vi "Enumerate Hardware.vi"(8 "error in (no error)":errorcluster, 11 "Hardware Info Module in":refnum<class "Hardware Info Module.lvclass">) -> (0 "error out":errorcluster, 3 "Hardware Info Module out":refnum<class "Hardware Info Module.lvclass">)   [LabVIEW 2023, in "Volatus.lvlib" / "Hardware Info Module.lvclass"]
uses:
  Hardware Info Module.lvclass
  HW Info.ctl
  <vilib>/nisyscfg/Close (Hardware).vi
  <vilib>/nisyscfg/Close (System).vi
  <vilib>/nisyscfg/nisyscfg.lvlib
  <resource>/objmgr/pxisysapi.rc
  <resource>/objmgr/nicriosae.rc
panel:
  out "Array":T1[](array[typedef])
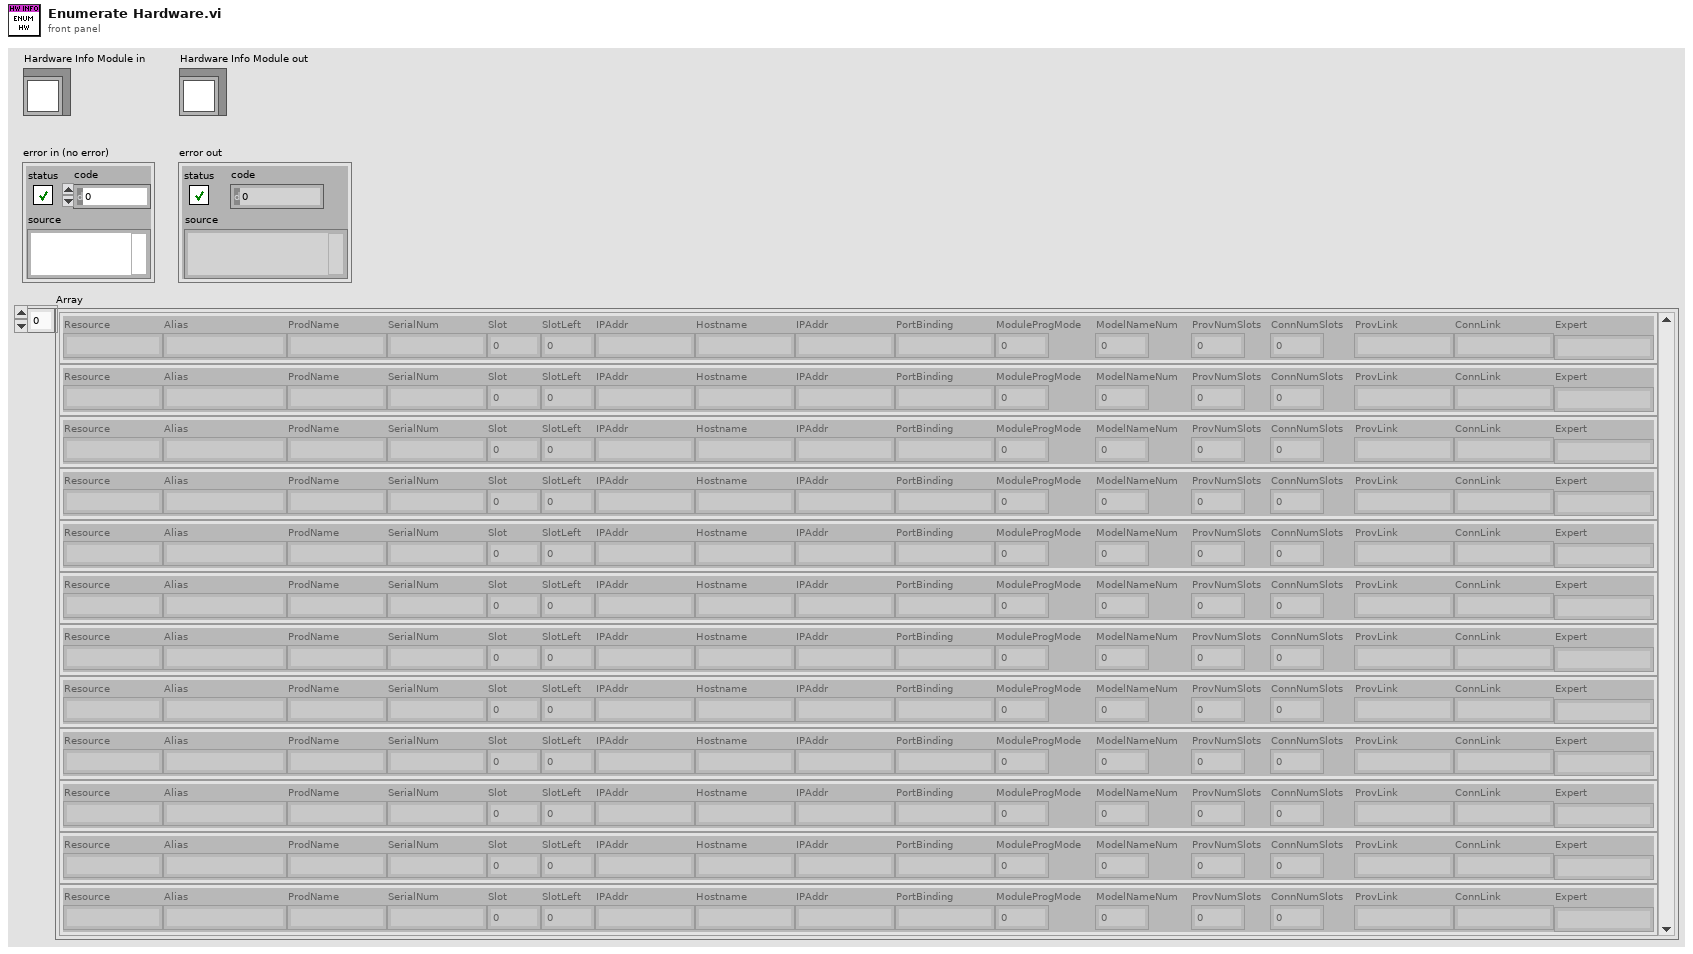
[diagram p1: front panel]
types:
  T1 = typedef "Volatus.lvlib/Hardware Info Module.lvclass/HW Info.ctl" = cluster{"Resource":string, "Alias":string, "ProdName":string, "SerialNum":string, "Slot":i32, "SlotLeft":u32, "IPAddr":string, "Hostname":string, "IPAddr":string, "PortBinding":string, "ModuleProgMode":u32, "ModelNameNum":u32, "ProvNumSlots":i32, "ConnNumSlots":i32, "ProvLink":string, "ConnLink":string, "Expert":string}
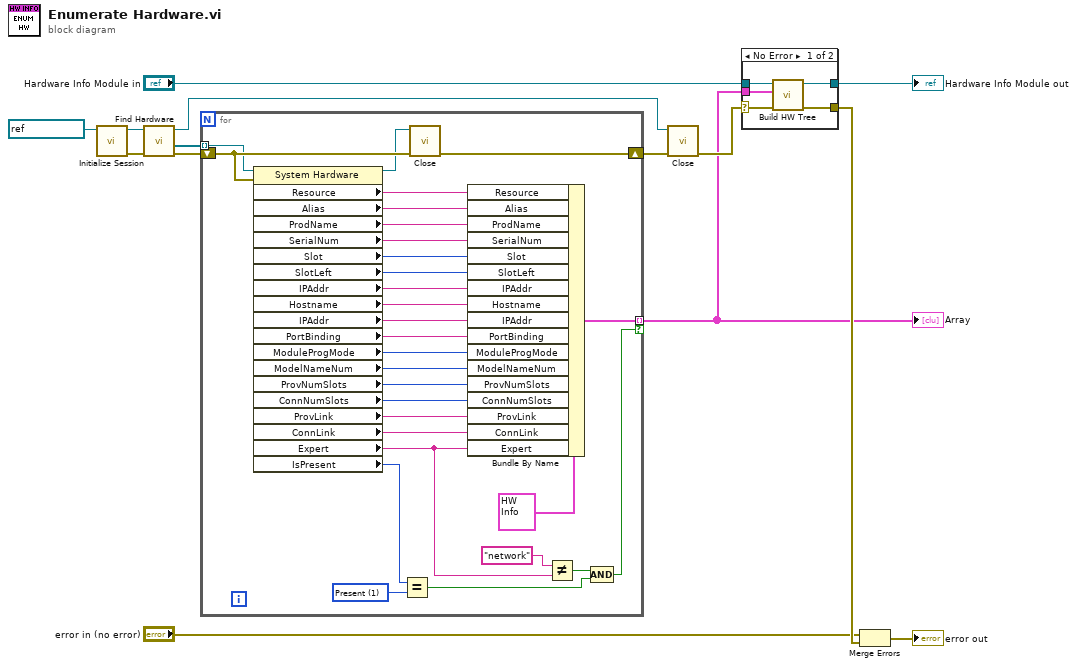
[diagram p0: block diagram]
diagram:
  n1 = call <vilib>:"Initialize Session.vi"("Target (localhost)"=refnum<k21> "localhost") -> ("error out"=w2:errorcluster, "Session out"=w3:refnum<k21>)  [unwired: 9 in]
  n2 = call <vilib>:"Find Hardware.vi"("error in (no error)"=w2, "Session in"=w3) -> ("error out"=w10:errorcluster, "Resources out"=w9:refnum<k20>[], "Session out"=w7:refnum<k21>)  [unwired: 6 in, 1 out]
  n3 = for {
    tunnel: w9 -> [w42] mode=indexing
    tunnel: [w17] -> w5 mode=indexing if=w36
    shift-right: [w34] -> w8
    shift-left: w10 -> [w43]
    w40 = 1 items=["Initializing"=-2, "Unknown"=-1, "Not Present"=0, "Present"=1] ("Devices & Chassis:Is Present")
    n4 = property class="System Hardware"(reference=w42, error in=w43) -> (reference out=w35:refnum<k20>, "Resource"=w16:string, "Alias"=w32:string, "ProdName"=w31:string, "SerialNum"=w30:string, "Slot"=w29:i32, "SlotLeft"=w28:u32, "IPAddr"=w27:string, "Hostname"=w26:string, "IPAddr"=w25:string, "PortBinding"=w24:string, "ModuleProgMode"=w23:u32, "ModelNameNum"=w22:u32, "ProvNumSlots"=w21:i32, "ConnNumSlots"=w20:i32, "ProvLink"=w19:string, "ConnLink"=w18:string, "Expert"=w15:string, "IsPresent"=w41:i32)  [unwired: 1 out]
    n5 = Equal?(x=w41, y=w40) -> (x = y?=w37:bool)
    n6 = call-poly <vilib>:"Close.vi"("error in (no error)"=w43, "Resource in"=w35) -> ("error out"=w34:errorcluster)  [unwired: 9 in]
    n7 = Bundle By Name(cluster=T1 {"Resource"="", "Alias"="", "ProdName"="", "SerialNum"="", "Slot"=0, "SlotLeft"=0, "IPAddr"="", "Hostname"="", "IPAddr"="", "PortBinding"="", "ModuleProgMode"=0, "ModelNameNum"=0, "ProvNumSlots"=0, "ConnNumSlots"=0, "ProvLink"="", "ConnLink"="", "Expert"=""} ("HW Info"), "Resource"=w16, "Alias"=w32, "ProdName"=w31, "SerialNum"=w30, "Slot"=w29, "SlotLeft"=w28, "IPAddr"=w27, "Hostname"=w26, "IPAddr"=w25, "PortBinding"=w24, "ModuleProgMode"=w23, "ModelNameNum"=w22, "ProvNumSlots"=w21, "ConnNumSlots"=w20, "ProvLink"=w19, "ConnLink"=w18, "Expert"=w15) -> (w17:T1)
    n8 = Not Equal?(x="network" ("y"), y=w15) -> (x != y?=w38:bool)
    n9 = Compound Arithmetic op=AND(w38, w37) -> (w36:bool)
  }
  "Array" <- w5
  n10 = call-poly <vilib>:"Close.vi"("error in (no error)"=w8, "Session in"=w7) -> ("error out"=w13:errorcluster)  [unwired: 9 in]
  n11 = case shown="No Error" w13 {
    selector: w13 -> [w45 w49]
    tunnel: "Hardware Info Module in" -> [w48 w50]
    tunnel: [w47 w50] -> w6
    tunnel: w5 -> [w46 _]
    tunnel: [w44 w49] -> w14
    frame No Error {
      n12 = call "Build HW Tree.vi"("error in (no error)"=w45, "HW Info"=w46, "Hardware Info Module in"=w48) -> ("error out"=w44:errorcluster, "Hardware Info Module out"=w47:refnum<class "Hardware Info Module.lvclass">)  [unwired: 7 in]
    }
    frame Error {
    }
  }
  "Hardware Info Module out" <- w6
  n13 = Merge Errors("error in (no error)", w14) -> (→"error out":errorcluster)
